vi "RF Rec Read FIFO (Two Channels).vi"(2 "fifo 0":refnum<k21>, 3 "fifo 1":refnum<k21>, 5 "enable":bool[](array[boolean]), 12 "ready for output":bool) -> (4 "data":u32[](array[numeric]), 10 "output valid":bool)   [LabVIEW 2018]
doc: "Reads data from two 32-bit FIFOs. This VI is a wrapper around the LabVIEW FPGA FIFO Read method. This VI exposes handshaking signals to control when data is read from the FIFOs.\n\n<B>Input Parameters</B>\n\n<B>enabled</B> specifies which streams are enabled.\n\n<B>fifo 0</B> is the reference to the FIFO which contains data to be sent over channel 0.\n\n<B>fifo 1</B> is the reference to the FIFO which contains data to be sent over channel 1.\n\n<B>ready for output</B> specifies whether the downstream node is ready for new data.\n\n<B>Output Parameters</B>\n\n<B>data out</B> is the data read from the FIFO and to be transmitted.\n\n<B>output valid</B> specifies when 'data out' is valid."
uses:
  <vilib>/rvi/DataTransferAndStorage/Container/Common/niFpgaContainerExecOnDevCompGetState.vi
  <vilib>/rvi/Emulation/niFpgaEmulationIsFPGAContextNoSignature.vi
  <vilib>/rvi/Emulation/niFpgaSctlEmulationGetInTimedLoop.vi
  <vilib>/rvi/errors/niFpgaSetErrorForExecOnDevCompSimple.vi
  <vilib>/rvi/eio/common/nirviEmuReportErrorAndStop.vi
  <vilib>/rvi/DataTransferAndStorage/Container/Common/niFpgaContainerGetUniqueNameForEmu.vi
  <vilib>/rvi/FIFO/Fifo_Resource/nirvififoEmulationSetSize.vi
  <vilib>/rvi/FIFO/Fifo_Resource/nirviFifoEmulationQueueMgr.vi
  <instcachedir>/0/nirviFifoEmulationQueueMgr_E5CAEC123FF24DC58D834DCA3CDAA9B5.lvgen/nirviFifoEmulationQueueMgr_E5CAEC123FF24DC58D834DCA3CDAA9B5_000.vi
  <vilib>/rvi/FIFO/Fifo_Resource/nirvififoEmulationDetermineInputValidOut.vi
  <vilib>/rvi/FIFO/Fifo_Resource/nirvififoEmulationCreateLock.vi
  <vilib>/rvi/Emulation/niFpgaProcessEmulError.vi
  <vilib>/rvi/FIFO/Fifo_Resource/nirvififoEmulationObtainLock.vi
  <vilib>/rvi/FIFO/Fifo_Resource/nirvififoEmulationReleaseLock.vi
  <vilib>/rvi/occurrence/nirviWaitOnOccurrenceBase.vi
  <vilib>/rvi/errors/nirviReportUnexpectedCaseInternalError.vi
  <vilib>/rvi/errors/nirviReportUnexpectedCaseInternalError (U32).vi
  <vilib>/Utility/error.llb/Clear Errors.vi
  <vilib>/rvi/interface/RandomDataEmulation/niFpgaRandomDataHandleErrors.vi
  <vilib>/rvi/DataTransferAndStorage/Container/XNode/niFpgaContainer.xnode
  <vilib>/rvi/FIFO/Fifo_Resource/niFpgaFifoEmulationRefIn.vi
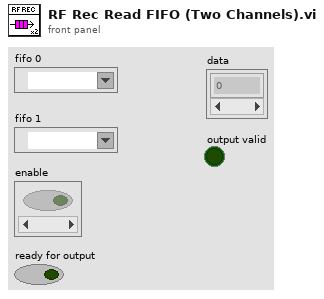
[diagram p1: front panel]
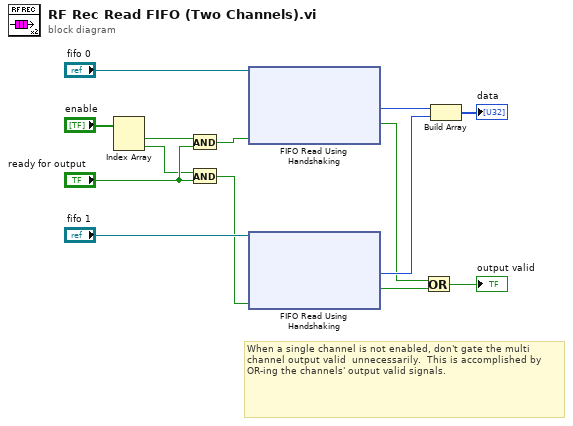
[diagram p0: block diagram]
diagram:
  # "When a single channel is not enabled, don't gate the multi channel output valid  unnecessarily.  This is accomplished by OR-ing the channels' output valid signals."
  n1 = Index Array(array="enable") -> (element #1=w14:bool, element #2=w10:bool)  [unwired: 2 in]
  n2 = And(x=w14, y="ready for output") -> (x .and. y?=w8:bool)
  n3 = And(x=w10, y="ready for output") -> (x .and. y?=w6:bool)
  n4 = xnode "FIFO Read Using Handshaking"("Ready for Output"=w8, "FIFO In"="fifo 0") -> ("Element"=w4:u32, "Output Valid"=w3:bool)  [unwired: 1 out]
  n5 = xnode "FIFO Read Using Handshaking"("Ready for Output"=w6, "FIFO In"="fifo 1") -> ("Element"=w5:u32, "Output Valid"=w2:bool)  [unwired: 1 out]
  n6 = Or(x=w3, y=w2) -> (x .or. y?=→"output valid":bool)
  n7 = Build Array(w4, w5) -> (→"data":u32[])
